vi "Call Subpanel VI.vi"(8 "error in (no error)":errorcluster, 10 "VI Refnum":refnum<vi>, 11 "VacuumLines Configuration in":refnum<class "VacuumLines Configuration.lvclass">) -> (0 "error out":errorcluster, 3 "VacuumLines Configuration out":refnum<class "VacuumLines Configuration.lvclass">)   [LabVIEW 2016, in "Hardware.lvlib" / "VacuumLine.lvlib" / "VacuumLines Configuration.lvclass"]
uses:
  <userlib>/Common Components/Hardware/Abstract System/VacuumLine/VacuumLines Configuration/VacuumLines Configuration.lvclass
  <userlib>/Configuration Dialog Actor/Configuration.lvclass
  C:/Program Files (x86)/National Instruments/LabVIEW 2016/user.lib/Configuration Dialog Actor/Configuration.lvclass
  <userlib>/Configuration Dialog Actor/Configuration.lvclass/Configuration.ctl
  <userlib>/Common Components/UserPwd DB/UserPwd DB Config/UserPwd DB Configuration.lvclass
  <userlib>/Common Components/Hardware/Abstract System/VacuumLine/VacuumLine Config/VacuumLine Configuration.lvclass
  <userlib>/Common Components/Hardware/Motor/Motor Config/Motor Configuration.lvclass
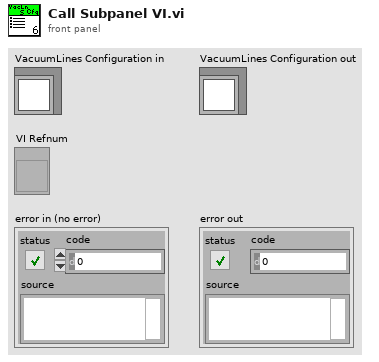
[diagram p1: front panel]
types:
  T1 = cluster{"Conflict Zones":string, "More Valves":string, "Pressure Display":string, "Temperature":string}
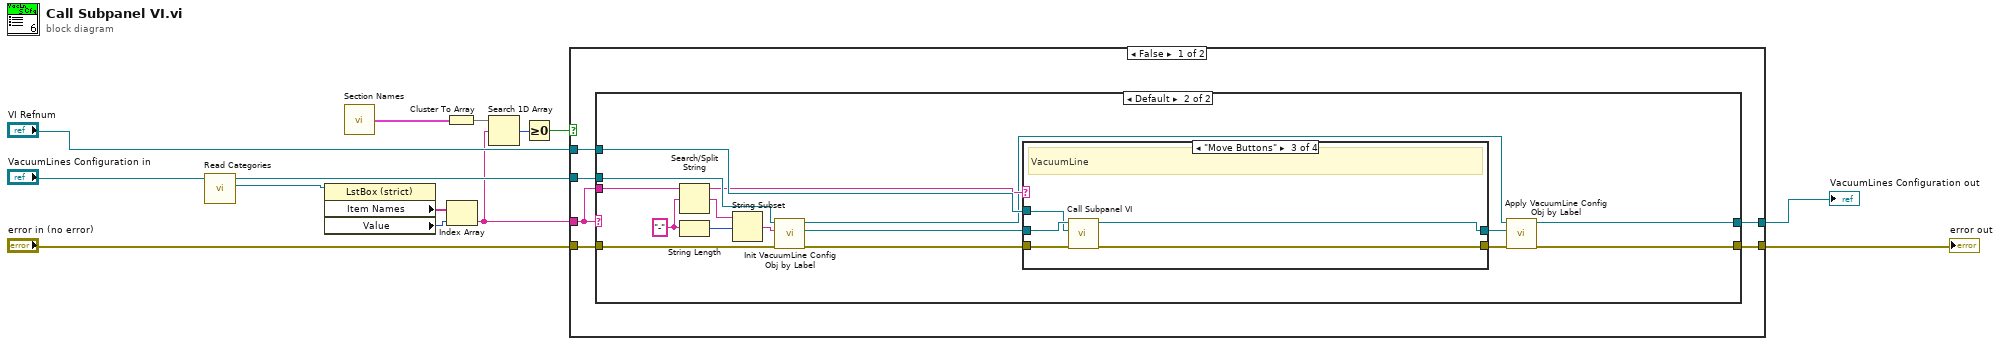
[diagram p0: block diagram]
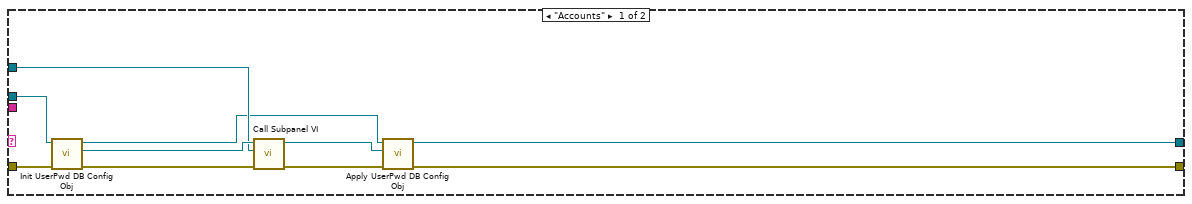
[diagram p2: hidden frame]
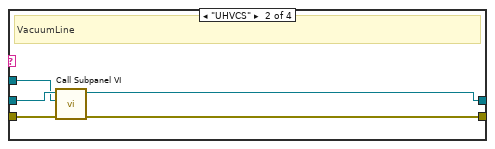
[diagram p4: hidden frame]
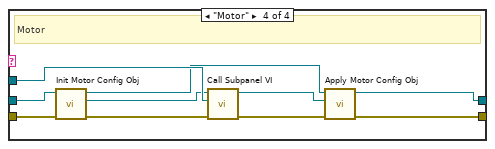
[diagram p5: hidden frame]
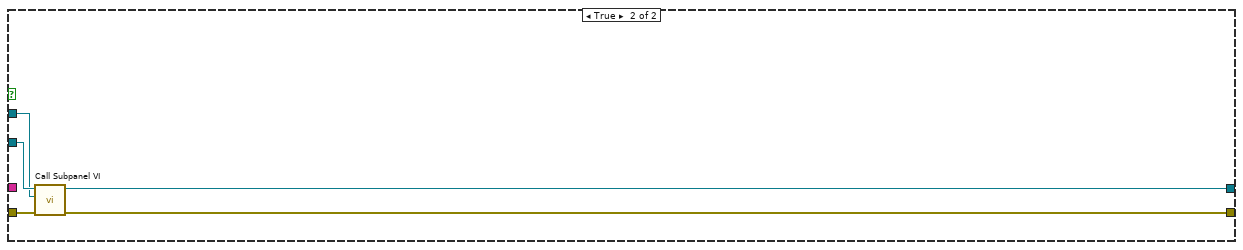
[diagram p6: hidden frame]
diagram:
  n1 = call <userlib>:"Read Categories.vi"("Configuration in"="VacuumLines Configuration in") -> ("Categories"=w14:refnum<vi>, "Configuration out"=w6:refnum<class "VacuumLines Configuration.lvclass">)  [unwired: 8 in, 1 out]
  n2 = property class="LstBox (strict)"(reference=w14) -> ("Item Names"=w7:string[], "Value"=w13:i32)  [unwired: 1 in, 2 out]
  n3 = call <userlib>:"Section Names.vi"() -> ("Cluster"=w5:T1)
  n4 = Cluster To Array(cluster=w5) -> (array=w4:string[])
  n5 = Index Array(array=w7, index=w13) -> (element=w3:string)
  n6 = Search 1D Array(1D array=w4, element=w3) -> (index of element=w2:i32)  [unwired: 1 in]
  n7 = Greater Or Equal To 0?(x=w2) -> (x >= 0?=w1:bool)
  n8 = case shown="False" w1 {
    tunnel: "VI Refnum" -> [w20 w69]
    tunnel: "error in (no error)" -> [w19 w73]
    tunnel: [w18 w72] -> w9
    tunnel: [w17 w70] -> w8
    tunnel: w6 -> [w16 w71]
    tunnel: w3 -> [w15 _]
    frame False {
      n9 = case shown="Default" w15 {
        tunnel: w20 -> [w25 w46]
        tunnel: w19 -> [w30 w45]
        tunnel: [w24 w42] -> w18
        tunnel: [w22 w41] -> w17
        tunnel: w16 -> [w28 w36]
        tunnel: w15 -> [_ w31]
        frame "Accounts" {
          n10 = call <userlib>:"Init UserPwd DB Config Obj.vi"("error in (no error)"=w30, "VacuumLines Configuration in"=w28) -> ("error out"=w29:errorcluster, "UserPwd DB Configuration Obj"=w26:refnum<class "UserPwd DB Configuration.lvclass">, "VacuumLines Configuration out"=w23:refnum<class "VacuumLines Configuration.lvclass">)  [unwired: 7 in]
          n11 = call-dynamic "Call Subpanel VI.vi"("error in (no error)"=w29, "VI Refnum"=w25, "UserPwd DB Configuration in"=w26) -> ("error out"=w27:errorcluster, "UserPwd DB Configuration out"=w21:refnum<class "UserPwd DB Configuration.lvclass">)  [unwired: 7 in]
          n12 = call <userlib>:"Apply UserPwd DB Config Obj.vi"("error in (no error)"=w27, "UserPwd DB Configuration Obj"=w21, "VacuumLines Configuration in"=w23) -> ("error out"=w24:errorcluster, "VacuumLines Configuration out"=w22:refnum<class "VacuumLines Configuration.lvclass">)  [unwired: 7 in]
        }
        frame Default {
          w32 = "-" ("search string/char (-)")
          n13 = Search/Split String(string=w31, search string/char (-)=w32) -> (substring before match=w35:string, match + rest of string=w39:string)  [unwired: 1 in, 1 out]
          n14 = String Length(string=w32) -> (length=w38:i32)
          n15 = String Subset(string=w39, offset (0)=w38) -> (substring=w37:string)  [unwired: 1 in]
          n16 = call <userlib>:"Init VacuumLine Config Obj by Label.vi"("error in (no error)"=w45, "label"=w37, "VacuumLines Configuration in"=w36) -> ("error out"=w43:errorcluster, "VacuumLine Configuration Obj"=w40:refnum<class "VacuumLine Configuration.lvclass">, "VacuumLines Configuration out"=w34:refnum<class "VacuumLines Configuration.lvclass">)  [unwired: 5 in, 1 out]
          n17 = case shown="\"Move Buttons\"" w35 {
            tunnel: [w47 w52 w57 w62] -> w44
            tunnel: [w48 w50 w55 w59] -> w33
            tunnel: w43 -> [w47 w53 w58 w66]
            tunnel: w46 -> [_ w49 w54 w68]
            tunnel: w40 -> [w48 w51 w56 w65]
            frame Default {
            }
            frame "UHVCS" {
              # "VacuumLine"
              n18 = call-dynamic "Call Subpanel VI.vi"("error in (no error)"=w53, "VI Refnum"=w49, "VacuumLine Configuration in"=w51) -> ("error out"=w52:errorcluster, "VacuumLine Configuration out"=w50:refnum<class "VacuumLine Configuration.lvclass">)  [unwired: 7 in]
            }
            frame "Move Buttons" {
              # "VacuumLine"
              n19 = call-dynamic "Call Subpanel VI.vi"("error in (no error)"=w58, "VI Refnum"=w54, "VacuumLine Configuration in"=w56) -> ("error out"=w57:errorcluster, "VacuumLine Configuration out"=w55:refnum<class "VacuumLine Configuration.lvclass">)  [unwired: 7 in]
            }
            frame "Motor" {
              # "Motor"
              n20 = call <userlib>:"Init Motor Config Obj.vi"("error in (no error)"=w66, "VacuumLine Configuration in"=w65) -> ("error out"=w64:errorcluster, "Motor Config Obj"=w63:refnum<class "Motor Configuration.lvclass">, "VacuumLine Configuration out"=w61:refnum<class "VacuumLine Configuration.lvclass">)  [unwired: 7 in]
              n21 = call-dynamic "Call Subpanel VI.vi"("error in (no error)"=w64, "VI Refnum"=w68, "Motor Configuration in"=w63) -> ("error out"=w67:errorcluster, "Motor Configuration out"=w60:refnum<class "Motor Configuration.lvclass">)  [unwired: 7 in]
              n22 = call <userlib>:"Apply Motor Config Obj.vi"("error in (no error)"=w67, "Motor Config Obj"=w60, "VacuumLine Configuration in"=w61) -> ("error out"=w62:errorcluster, "VacuumLine Configuration out"=w59:refnum<class "VacuumLine Configuration.lvclass">)  [unwired: 7 in]
            }
          }
          n23 = call <userlib>:"Apply VacuumLine Config Obj by Label.vi"("error in (no error)"=w44, "VacuumLine Configuration Obj"=w33, "VacuumLines Configuration in"=w34) -> ("error out"=w42:errorcluster, "VacuumLines Configuration out"=w41:refnum<class "VacuumLines Configuration.lvclass">)  [unwired: 7 in]
        }
      }
    }
    frame True {
      n24 = call-parent "Call Subpanel VI.vi"("error in (no error)"=w73, "VI Refnum"=w69, "Configuration in"=w71) -> ("error out"=w72:errorcluster, "Configuration out"=w70:refnum<class "VacuumLines Configuration.lvclass">)  [unwired: 7 in]
    }
  }
  "error out" <- w9
  "VacuumLines Configuration out" <- w8
